vi "Reverse Sort Test.vi"(11 "Error In":errorcluster) -> (15 "Error Out":errorcluster)   [LabVIEW 2021, in "Test Files.lvlib"]
doc: "This VI has test cases for checking sorting array in reverse order."
uses:
  Test Files.lvlib
  <vilib>/addons/_JKI Toolkits/Caraya/classes/Test/Test.lvclass
  <vilib>/addons/_JKI Toolkits/Caraya/classes/Assert/Assert.lvclass
  CustomSortPath.lvlib
  <vilib>/addons/_JKI Toolkits/Caraya/classes/Assert/Assert Equal Value_Variant.vi
panel:
  # "Sort in reverse(Z to A) order test"
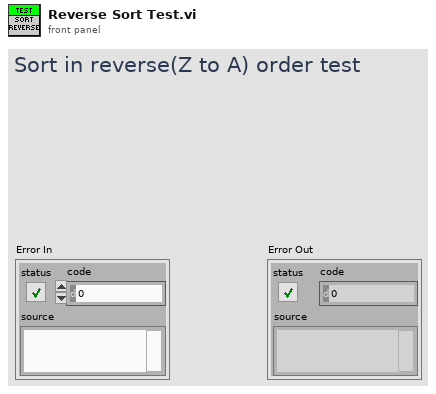
[diagram p1: front panel]
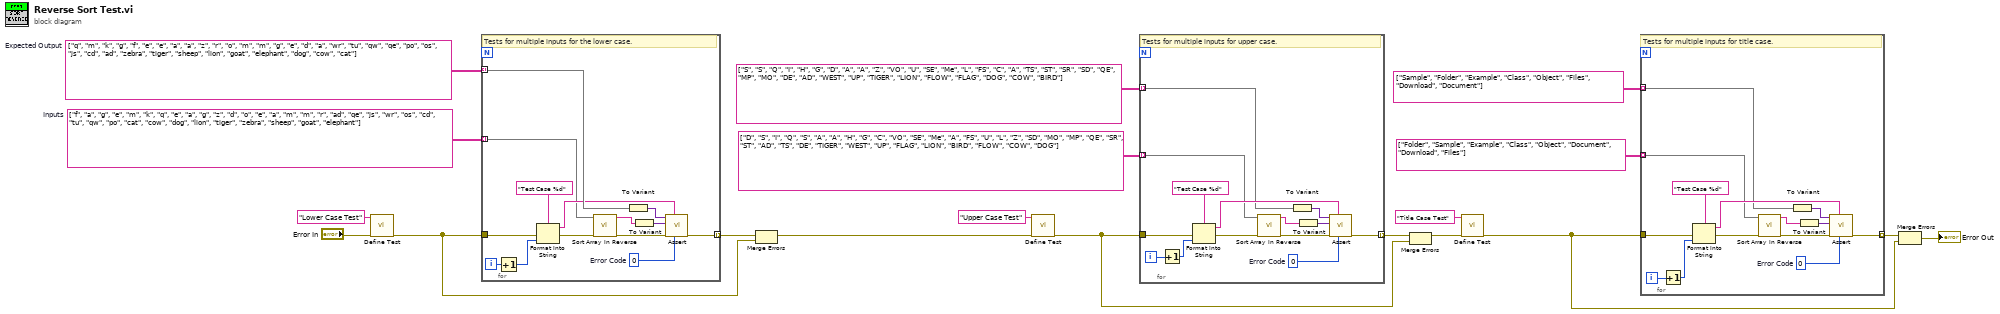
[diagram p0: block diagram]
diagram:
  w16 = string[][] [["q", "m", "k", "g", "f", "e", "e", "a", "a"], ["z", "r", "o", "m", "m", "g", "e", "d", "a"], ["wr", "tu", "qw", "qe", "po", "os", "js", "cd", "ad"], ["zebra", "tiger", "sheep", "lion", "goat", "elephant", "dog", "cow", "cat"]]  # Expected Output
  w17 = string[][] [["f", "a", "g", "e", "m", "k", "q", "e", "a"], ["g", "z", "d", "o", "e", "a", "m", "m", "r"], ["ad", "qe", "js", "wr", "os", "cd", "tu", "qw", "po"], ["cat", "cow", "dog", "lion", "tiger", "zebra", "sheep", "goat", "elephant"]]  # Inputs
  n1 = call <vilib>:"Define Test.vi"("error in (no error)"="Error In", "Label (VI Title)"="Lower Case Test") -> ("error out"=w7:errorcluster)  [unwired: 8 in, 1 out]
  n2 = for {
    tunnel: w17 -> [w22] mode=indexing
    tunnel: w16 -> [w26] mode=indexing
    tunnel: w7 -> [w32]
    tunnel: [w33] -> w9 mode=indexing
    i -> [w30]
    w20 = 0  # Error Code
    # "Tests for multiple inputs for the lower case."
    n3 = Increment(x=w30) -> (x+1=w21:i32)
    n4 = Format Into String(format string="Test Case %d", error in=w32, w21) -> (resulting string=w24:string, error out=w29:errorcluster)  [unwired: 1 in]
    n5 = call "Sort Array In Reverse.vi"("InputArray"=w22, "error in (no error)"=w29) -> ("SortedArray"=w23:string[], "error out"=w28:errorcluster)  [unwired: 12 in]
    n6 = To Variant(anything=w26) -> (Variant=w25:variant)
    n7 = To Variant(anything=w23) -> (Variant=w27:variant)
    n8 = call-poly <vilib>:"Assert.vi"("error code (1)"=w20, "Label"=w24, "error in (no error)"=w28, "Y"=w27, "X"=w25) -> ("error out"=w33:errorcluster)  [unwired: 5 in, 1 out]
  }
  n9 = Merge Errors(w9, w7) -> (w8:errorcluster)
  n10 = call <vilib>:"Define Test.vi"("error in (no error)"=w8, "Label (VI Title)"="Upper Case Test") -> ("error out"=w4:errorcluster)  [unwired: 8 in, 1 out]
  n11 = for {
    tunnel: string[][] [["D", "S", "I", "Q", "S", "A", "A", "H", "G"], ["C", "VO", "SE", "Me", "A", "FS", "U", "L", "Z"], ["SD", "MO", "MP", "QE", "SR", "ST", "AD", "TS", "DE"], ["TIGER", "WEST", "UP", "FLAG", "LION", "BIRD", "FLOW", "COW", "DOG"]] ("appended array") -> [w38] mode=indexing
    tunnel: string[][] [["S", "S", "Q", "I", "H", "G", "D", "A", "A"], ["Z", "VO", "U", "SE", "Me", "L", "FS", "C", "A"], ["TS", "ST", "SR", "SD", "QE", "MP", "MO", "DE", "AD"], ["WEST", "UP", "TIGER", "LION", "FLOW", "FLAG", "DOG", "COW", "BIRD"]] ("appended array") -> [w37] mode=indexing
    tunnel: w4 -> [w46]
    tunnel: [w47] -> w6 mode=indexing
    i -> [w44]
    w34 = 0  # Error Code
    # "Tests for multiple inputs for upper case."
    n12 = Increment(x=w44) -> (x+1=w35:i32)
    n13 = Format Into String(format string="Test Case %d", error in=w46, w35) -> (resulting string=w39:string, error out=w43:errorcluster)  [unwired: 1 in]
    n14 = call "Sort Array In Reverse.vi"("InputArray"=w38, "error in (no error)"=w43) -> ("SortedArray"=w36:string[], "error out"=w42:errorcluster)  [unwired: 12 in]
    n15 = To Variant(anything=w37) -> (Variant=w40:variant)
    n16 = To Variant(anything=w36) -> (Variant=w41:variant)
    n17 = call-poly <vilib>:"Assert.vi"("error code (1)"=w34, "Label"=w39, "error in (no error)"=w42, "Y"=w41, "X"=w40) -> ("error out"=w47:errorcluster)  [unwired: 5 in, 1 out]
  }
  n18 = Merge Errors(w6, w4) -> (w5:errorcluster)
  n19 = call <vilib>:"Define Test.vi"("error in (no error)"=w5, "Label (VI Title)"="Title Case Test") -> ("error out"=w1:errorcluster)  [unwired: 8 in, 1 out]
  n20 = for {
    tunnel: string[][] [["Folder", "Sample", "Example", "Class"], ["Object", "Document", "Download", "Files"]] ("appended array") -> [w52] mode=indexing
    tunnel: string[][] [["Sample", "Folder", "Example", "Class"], ["Object", "Files", "Download", "Document"]] ("appended array") -> [w51] mode=indexing
    tunnel: w1 -> [w60]
    tunnel: [w61] -> w2 mode=indexing
    i -> [w58]
    w48 = 0  # Error Code
    # "Tests for multiple inputs for title case."
    n21 = Increment(x=w58) -> (x+1=w49:i32)
    n22 = Format Into String(format string="Test Case %d", error in=w60, w49) -> (resulting string=w53:string, error out=w57:errorcluster)  [unwired: 1 in]
    n23 = call "Sort Array In Reverse.vi"("InputArray"=w52, "error in (no error)"=w57) -> ("SortedArray"=w50:string[], "error out"=w56:errorcluster)  [unwired: 12 in]
    n24 = To Variant(anything=w51) -> (Variant=w54:variant)
    n25 = To Variant(anything=w50) -> (Variant=w55:variant)
    n26 = call-poly <vilib>:"Assert.vi"("error code (1)"=w48, "Label"=w53, "error in (no error)"=w56, "Y"=w55, "X"=w54) -> ("error out"=w61:errorcluster)  [unwired: 5 in, 1 out]
  }
  n27 = Merge Errors(w2, w1) -> (→"Error Out":errorcluster)
